vi "Manage Server Attribute.vi"(0 "All Interfaces Dict in":variant, 2 "Specific Interface Dict in":variant, 3 "Message Enqueuer in":refnum<class "Message Enqueuer.lvclass">, 4 "Listener Settings":T1, 5 "error in (no error)":errorcluster, 8 "Is \"All Interface\" Server":bool, 9 "Action":enum16{"Set", "Get", "Delete"}(ring)) -> (14 "All Interfaces Dict out":variant, 16 "Specific Interface Dict out":variant, 17 "Message Enqueuer out":refnum<class "Message Enqueuer.lvclass">, 19 "error out":errorcluster)   [LabVIEW 2016, in "WebSocket Actors.lvlib" / "WebSocket Server Manager.lvclass"]
uses:
  WebSocket Server Manager.lvclass
  <vilib>/ActorFramework/Message Enqueuer/Message Enqueuer.lvclass
  WebSocket Server/typedefs/Listener Settings.ctl
  WebSocket Server/WebSocket Server.lvclass
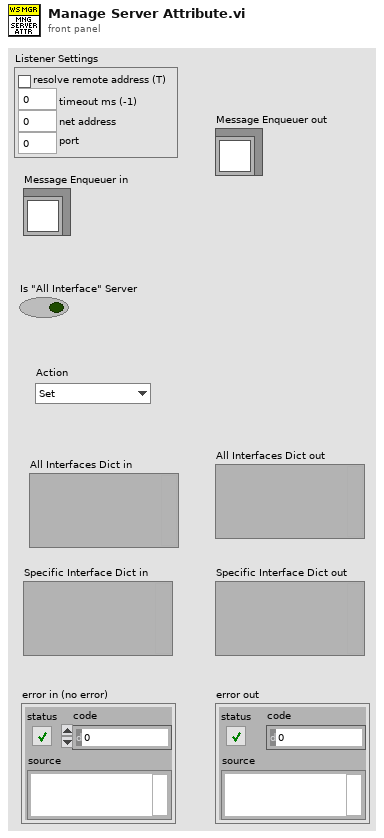
[diagram p1: front panel]
types:
  T1 = typedef "WebSocket Actors.lvlib/WebSocket Server.lvclass/Listener Settings.ctl" = cluster{"resolve remote address (T)":bool, "timeout ms (-1)":i32, "net address":u32, "port":u16}
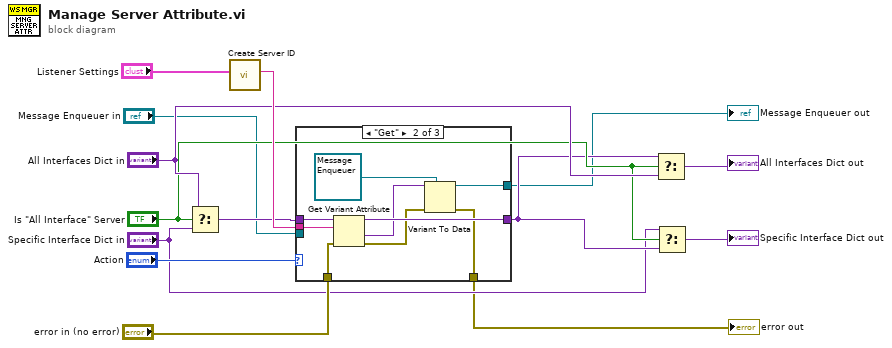
[diagram p0: block diagram]
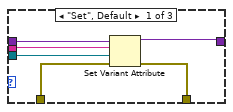
[diagram p2: hidden frame]
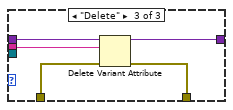
[diagram p3: hidden frame]
diagram:
  n1 = Select(t="All Interfaces Dict in", s="Is \"All Interface\" Server", f="Specific Interface Dict in") -> (s? t:f=w10:variant)
  n2 = call "Create Server ID.vi"("Listener Settings"="Listener Settings") -> ("Server URI"=w14:string)  [unwired: 7 in, 2 out]
  n3 = case shown="\"Get\"" "Action" {
    tunnel: w10 -> [w19 w29 w32]
    tunnel: [w18 w28 w31] -> w6
    tunnel: "error in (no error)" -> [w20 w27 w33]
    tunnel: [w17 w22 w34] -> w2
    tunnel: w14 -> [w16 w26 w30]
    tunnel: "Message Enqueuer in" -> [w15 _ _]
    tunnel: [_ w21 _] -> w1
    frame "Set", Default {
      n4 = Set Variant Attribute(Variant=w19, name=w16, value=w15, error in=w20) -> (Variant out=w18:variant, error out=w17:errorcluster)  [unwired: 1 out]
    }
    frame "Get" {
      n5 = Get Variant Attribute(Variant=w29, name=w26, error in=w27) -> (duplicate Variant=w28:variant, value=w23:variant, error out=w24:errorcluster)  [unwired: 1 in, 1 out]
      n6 = Variant To Data(error in=w24, type=refnum<class "Message Enqueuer.lvclass"> refnum ("Nested Actor's Enqueuer"), Variant=w23) -> (data=w21:refnum<class "Message Enqueuer.lvclass">, error out=w22:errorcluster)
    }
    frame "Delete" {
      n7 = Delete Variant Attribute(4:w33, 6:w30, 7:w32) -> (0:w34:errorcluster, 3:w31:variant)  [unwired: 1 out]
    }
  }
  "Message Enqueuer out" <- w1
  "error out" <- w2
  n8 = Select(t=w6, s="Is \"All Interface\" Server", f="All Interfaces Dict in") -> (s? t:f=→"All Interfaces Dict out":variant)
  n9 = Select(t="Specific Interface Dict in", s="Is \"All Interface\" Server", f=w6) -> (s? t:f=→"Specific Interface Dict out":variant)
